vi "Check Switch Schedule.vi"(8 "error in (no error)":errorcluster, 11 "Switch Schedule":T4) -> (0 "error out":errorcluster, 1 "Switch Program":T1, 2 "Trigger?":bool, 3 "On/Off":bool)   [LabVIEW 2014]
doc: "Compares the current time to the switch schedule and outputs a boolean to indicate if a switch program has been triggered."
uses:
  myRIO/Controls/Switch Schedule.ctl
  myRIO/Controls/Switch Program.ctl
  myRIO/Controls/Action Enum.ctl
  myRIO/Controls/Switch Day.ctl
panel:
  out "Action":T2
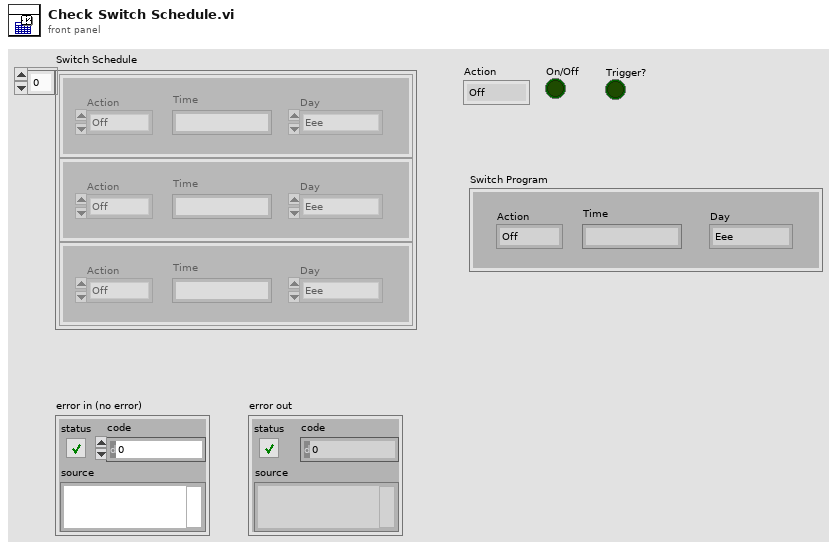
[diagram p1: front panel]
types:
  T1 = typedef "Switch Program.ctl" = cluster{"Action":T2, "Time":string, "Day":T3}
  T2 = typedef "Action Enum.ctl" = enum16{"Off", "On"}
  T3 = typedef "Switch Day.ctl" = enum16{"Eee", "Sun", "Mon", "Tue", "Wed", "Thu", "Fri", "Sat"}
  T4 = typedef "Switch Schedule.ctl" = T1[]
  T5 = typedef "LVDateTimeRec.ctl" = cluster{"fractional second":dbl, "second":i32, "minute":i32, "hour":i32, "day of month":i32, "month":i32, "year":i32, "day of week":i32, "day of year":i32, "DST":i32}
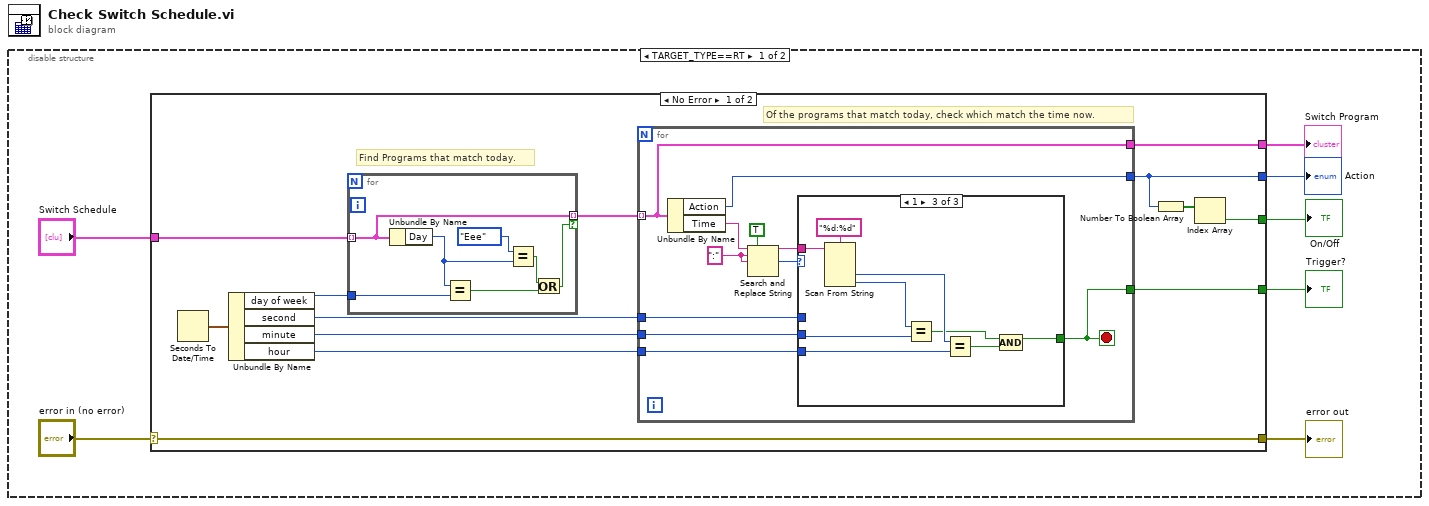
[diagram p0: block diagram]
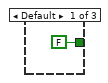
[diagram p2: hidden frame]
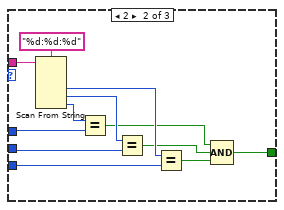
[diagram p3: hidden frame]
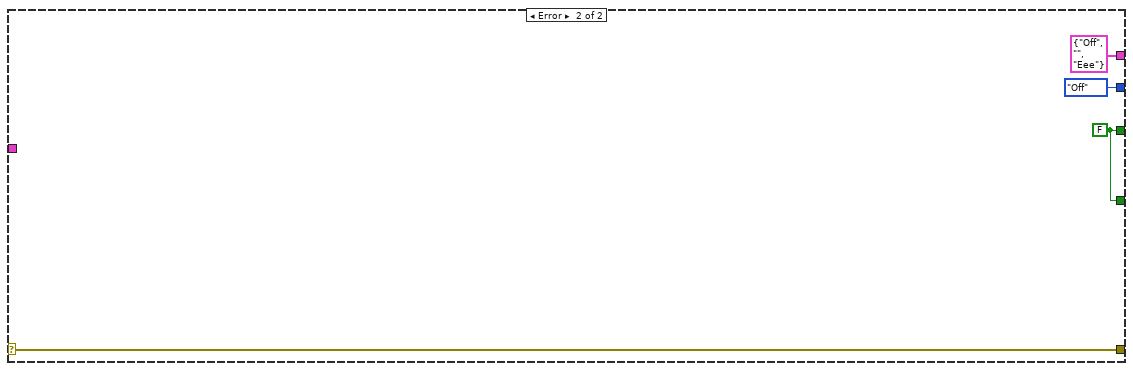
[diagram p4: hidden frame]
diagram:
  n1 = disable-structure shown="TARGET_TYPE==RT" {
    frame condition #0 (active) {
      n2 = case shown="No Error" "error in (no error)" {
        selector: "error in (no error)" -> [w10 w64]
        tunnel: "Switch Schedule" -> [w20 _]
        tunnel: [w12 w63] -> w6
        tunnel: [w11 w63] -> w5
        tunnel: [w10 w64] -> w3
        tunnel: [w9 Action_Enum."Off" ("Action")] -> w2
        tunnel: [w8 T1 {"Action"=enum."Off", "Time"="", "Day"=enum."Eee"} ("Switch Program")] -> w1
        frame No Error {
          # "Of the programs that match today, check which match the time now."
          # "Find Programs that match today."
          n3 = Seconds To Date/Time() -> (date time rec=w19:T5)  [unwired: 2 in]
          n4 = Unbundle By Name(w19) -> ("day of week"=w18:i32, "second"=w16:i32, "minute"=w15:i32, "hour"=w14:i32)
          n5 = for {
            tunnel: w20 -> [w59] mode=indexing
            tunnel: w18 -> [w60]
            tunnel: [w59] -> w17 mode=indexing if=w54
            n6 = Unbundle By Name(w59) -> ("Day"=w58:T3)
            n7 = Equal?(x=w58, y=w60) -> (x = y?=w55:bool)
            n8 = Equal?(x=Switch_Day."Eee" ("Day"), y=w58) -> (x = y?=w56:bool)
            n9 = Or(x=w56, y=w55) -> (x .or. y?=w54:bool)
          }
          n10 = for {
            tunnel: w17 -> [w21] mode=indexing
            tunnel: w16 -> [w24]
            tunnel: w15 -> [w26]
            tunnel: w14 -> [w25]
            tunnel: [w23] -> w9
            tunnel: [w22] -> w11
            tunnel: [w21] -> w8
            stop <- w22 stop-if-true
            w29 = ":" ("search string")
            n11 = Unbundle By Name(w21) -> ("Action"=w23:T2, "Time"=w31:string)
            n12 = Search and Replace String(replace all?=TRUE ("replace all? (F)"), input string=w31, search string=w29, replace string=w29) -> (result string=w27:string, number of replacements=w28:i32)  [unwired: 4 in, 2 out]
            n13 = case shown="1" w28 {
              tunnel: w27 -> [_ w43 w52]
              tunnel: w26 -> [_ w39 w50]
              tunnel: w25 -> [_ w38 w49]
              tunnel: w24 -> [_ w41 _]
              tunnel: [FALSE w33 w45] -> w22
              frame Default {
              }
              frame 2 {
                n14 = Scan From String(format string="%d:%d:%d", input string=w43) -> (output 1=w37:i32, output 2=w40:i32, output 3=w42:i32)  [unwired: 5 in, 3 out]
                n15 = Equal?(x=w42, y=w41) -> (x = y?=w34:bool)
                n16 = Equal?(x=w40, y=w39) -> (x = y?=w35:bool)
                n17 = Equal?(x=w37, y=w38) -> (x = y?=w36:bool)
                n18 = Compound Arithmetic op=AND(w34, w35, w36) -> (w33:bool)
              }
              frame 1 {
                n19 = Scan From String(format string="%d:%d", input string=w52) -> (output 1=w48:i32, output 2=w51:i32)  [unwired: 4 in, 3 out]
                n20 = Equal?(x=w51, y=w50) -> (x = y?=w46:bool)
                n21 = Equal?(x=w48, y=w49) -> (x = y?=w47:bool)
                n22 = Compound Arithmetic op=AND(w46, w47) -> (w45:bool)
              }
            }
          }
          n23 = Number To Boolean Array(number=w9) -> (Boolean array=w13:bool[])
          n24 = Index Array(array=w13) -> (element=w12:bool)  [unwired: 1 in]
        }
        frame Error {
          w63 = FALSE
        }
      }
      "On/Off" <- w6
      "Trigger?" <- w5
      "error out" <- w3
      "Action" <- w2
      "Switch Program" <- w1
    }
    frame condition #1 {
    }
  }
